vi "StorePreviousSwitchValues.vi"(0 "Array":u8[](array[numeric])) -> ()   [LabVIEW 2018]
uses:
  CurrentSwitchValues_GlobalVariable.vi
panel:
  out "30":dbl
  out "29":dbl
  out "28":dbl
  out "27":dbl
  out "26":dbl
  out "25":dbl
  out "24":dbl
  out "23":dbl
  out "22":dbl
  out "21":dbl
  out "20":dbl
  out "19":dbl
  out "18":dbl
  out "17":dbl
  out "16":dbl
  out "15":dbl
  out "14":dbl
  out "13":dbl
  out "12":dbl
  out "11":dbl
  out "10":dbl
  out "9":dbl
  out "8":dbl
  out "7":dbl
  out "6":dbl
  out "5":dbl
  out "4":dbl
  out "3":dbl
  out "2":dbl
  out "1":dbl
  out "[3]":string
  out "[4]":string
  out "[1]":string
  out "[2]":string
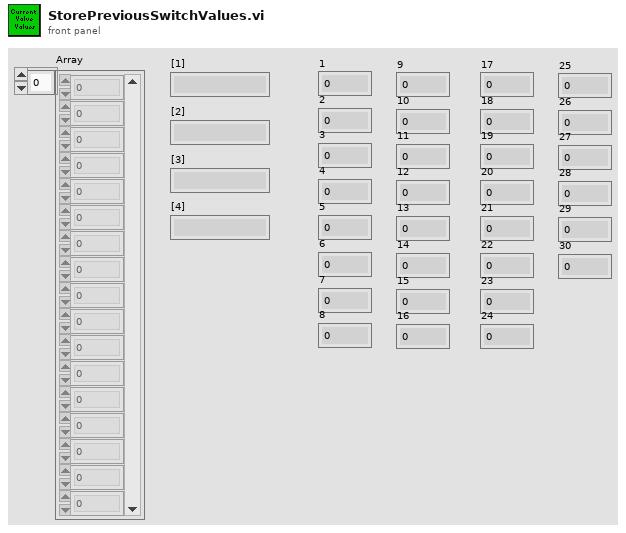
[diagram p1: front panel]
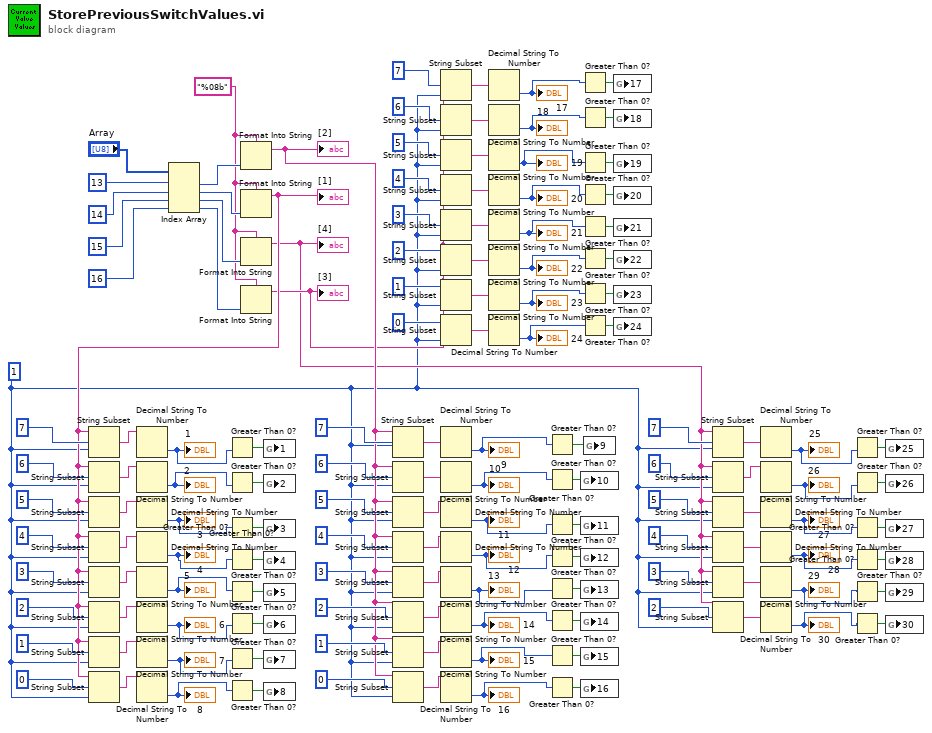
[diagram p0: block diagram]
diagram:
  w1 = 1
  w110 = "%08b"
  n1 = Index Array(array="Array", index #1=13, index #2=14, index #3=15, index #4=16) -> (element #1=w130:u8, element #2=w127:u8, element #3=w128:u8, element #4=w129:u8)
  n2 = Format Into String(format string=w110, w130) -> (resulting string=w93:string)  [unwired: 2 in, 1 out]
  "[2]" <- w93
  n3 = Format Into String(format string=w110, w127) -> (resulting string=w92:string)  [unwired: 2 in, 1 out]
  "[1]" <- w92
  n4 = String Subset(string=w92, offset (0)=7, length (rest)=w1) -> (substring=w126:string)
  n5 = String Subset(string=w92, offset (0)=6, length (rest)=w1) -> (substring=w119:string)
  n6 = String Subset(string=w92, offset (0)=5, length (rest)=w1) -> (substring=w120:string)
  n7 = String Subset(string=w92, offset (0)=4, length (rest)=w1) -> (substring=w121:string)
  n8 = String Subset(string=w92, offset (0)=3, length (rest)=w1) -> (substring=w122:string)
  n9 = String Subset(string=w92, offset (0)=2, length (rest)=w1) -> (substring=w123:string)
  n10 = String Subset(string=w92, offset (0)=1, length (rest)=w1) -> (substring=w124:string)
  n11 = String Subset(string=w92, offset (0)=0, length (rest)=w1) -> (substring=w125:string)
  n12 = Decimal String To Number(string=w126) -> (number=w61:i32)  [unwired: 2 in, 1 out]
  "1" <- w61
  n13 = Decimal String To Number(string=w119) -> (number=w46:i32)  [unwired: 2 in, 1 out]
  "2" <- w46
  n14 = Decimal String To Number(string=w120) -> (number=w47:i32)  [unwired: 2 in, 1 out]
  "3" <- w47
  n15 = Decimal String To Number(string=w121) -> (number=w48:i32)  [unwired: 2 in, 1 out]
  "4" <- w48
  n16 = Decimal String To Number(string=w122) -> (number=w49:i32)  [unwired: 2 in, 1 out]
  "5" <- w49
  n17 = Decimal String To Number(string=w123) -> (number=w50:i32)  [unwired: 2 in, 1 out]
  "6" <- w50
  n18 = Decimal String To Number(string=w124) -> (number=w51:i32)  [unwired: 2 in, 1 out]
  "7" <- w51
  n19 = Decimal String To Number(string=w125) -> (number=w52:i32)  [unwired: 2 in, 1 out]
  "8" <- w52
  n20 = Greater Than 0?(x=w61) -> (x > 0?=w60:bool)
  n21 = Greater Than 0?(x=w46) -> (x > 0?=w59:bool)
  n22 = Greater Than 0?(x=w47) -> (x > 0?=w58:bool)
  n23 = Greater Than 0?(x=w48) -> (x > 0?=w57:bool)
  n24 = Greater Than 0?(x=w49) -> (x > 0?=w56:bool)
  n25 = Greater Than 0?(x=w50) -> (x > 0?=w55:bool)
  n26 = Greater Than 0?(x=w51) -> (x > 0?=w54:bool)
  n27 = Greater Than 0?(x=w52) -> (x > 0?=w53:bool)
  n28 = Format Into String(format string=w110, w128) -> (resulting string=w63:string)  [unwired: 2 in, 1 out]
  "[4]" <- w63
  n29 = Format Into String(format string=w110, w129) -> (resulting string=w75:string)  [unwired: 2 in, 1 out]
  "[3]" <- w75
  n30 = global write "CurrentSwitchValues_GlobalVariable.vi" "1"(w60) -> ()
  n31 = global write "CurrentSwitchValues_GlobalVariable.vi" "2"(w59) -> ()
  n32 = global write "CurrentSwitchValues_GlobalVariable.vi" "3"(w58) -> ()
  n33 = global write "CurrentSwitchValues_GlobalVariable.vi" "4"(w57) -> ()
  n34 = global write "CurrentSwitchValues_GlobalVariable.vi" "5"(w56) -> ()
  n35 = global write "CurrentSwitchValues_GlobalVariable.vi" "6"(w55) -> ()
  n36 = global write "CurrentSwitchValues_GlobalVariable.vi" "7"(w54) -> ()
  n37 = global write "CurrentSwitchValues_GlobalVariable.vi" "8"(w53) -> ()
  n38 = String Subset(string=w93, offset (0)=7, length (rest)=w1) -> (substring=w109:string)
  n39 = String Subset(string=w93, offset (0)=6, length (rest)=w1) -> (substring=w102:string)
  n40 = String Subset(string=w93, offset (0)=5, length (rest)=w1) -> (substring=w103:string)
  n41 = String Subset(string=w93, offset (0)=4, length (rest)=w1) -> (substring=w104:string)
  n42 = String Subset(string=w93, offset (0)=3, length (rest)=w1) -> (substring=w105:string)
  n43 = String Subset(string=w93, offset (0)=2, length (rest)=w1) -> (substring=w106:string)
  n44 = String Subset(string=w93, offset (0)=1, length (rest)=w1) -> (substring=w107:string)
  n45 = String Subset(string=w93, offset (0)=0, length (rest)=w1) -> (substring=w108:string)
  n46 = String Subset(string=w75, offset (0)=7, length (rest)=w1) -> (substring=w91:string)
  n47 = String Subset(string=w75, offset (0)=6, length (rest)=w1) -> (substring=w84:string)
  n48 = String Subset(string=w75, offset (0)=5, length (rest)=w1) -> (substring=w85:string)
  n49 = String Subset(string=w75, offset (0)=4, length (rest)=w1) -> (substring=w86:string)
  n50 = String Subset(string=w75, offset (0)=3, length (rest)=w1) -> (substring=w87:string)
  n51 = String Subset(string=w75, offset (0)=2, length (rest)=w1) -> (substring=w88:string)
  n52 = String Subset(string=w75, offset (0)=1, length (rest)=w1) -> (substring=w89:string)
  n53 = String Subset(string=w75, offset (0)=0, length (rest)=w1) -> (substring=w90:string)
  n54 = Decimal String To Number(string=w109) -> (number=w21:i32)  [unwired: 2 in, 1 out]
  "9" <- w21
  n55 = Decimal String To Number(string=w102) -> (number=w20:i32)  [unwired: 2 in, 1 out]
  "10" <- w20
  n56 = Decimal String To Number(string=w103) -> (number=w19:i32)  [unwired: 2 in, 1 out]
  "11" <- w19
  n57 = Decimal String To Number(string=w104) -> (number=w18:i32)  [unwired: 2 in, 1 out]
  "12" <- w18
  n58 = Decimal String To Number(string=w105) -> (number=w17:i32)  [unwired: 2 in, 1 out]
  "13" <- w17
  n59 = Decimal String To Number(string=w106) -> (number=w16:i32)  [unwired: 2 in, 1 out]
  "14" <- w16
  n60 = Decimal String To Number(string=w107) -> (number=w15:i32)  [unwired: 2 in, 1 out]
  "15" <- w15
  n61 = Decimal String To Number(string=w108) -> (number=w14:i32)  [unwired: 2 in, 1 out]
  "16" <- w14
  n62 = Decimal String To Number(string=w91) -> (number=w22:i32)  [unwired: 2 in, 1 out]
  "17" <- w22
  n63 = Decimal String To Number(string=w84) -> (number=w23:i32)  [unwired: 2 in, 1 out]
  "18" <- w23
  n64 = Decimal String To Number(string=w85) -> (number=w24:i32)  [unwired: 2 in, 1 out]
  "19" <- w24
  n65 = Decimal String To Number(string=w86) -> (number=w25:i32)  [unwired: 2 in, 1 out]
  "20" <- w25
  n66 = Decimal String To Number(string=w87) -> (number=w26:i32)  [unwired: 2 in, 1 out]
  "21" <- w26
  n67 = Decimal String To Number(string=w88) -> (number=w27:i32)  [unwired: 2 in, 1 out]
  "22" <- w27
  n68 = Decimal String To Number(string=w89) -> (number=w28:i32)  [unwired: 2 in, 1 out]
  "23" <- w28
  n69 = Decimal String To Number(string=w90) -> (number=w29:i32)  [unwired: 2 in, 1 out]
  "24" <- w29
  n70 = Greater Than 0?(x=w21) -> (x > 0?=w38:bool)
  n71 = Greater Than 0?(x=w20) -> (x > 0?=w39:bool)
  n72 = Greater Than 0?(x=w19) -> (x > 0?=w40:bool)
  n73 = Greater Than 0?(x=w18) -> (x > 0?=w41:bool)
  n74 = Greater Than 0?(x=w17) -> (x > 0?=w42:bool)
  n75 = Greater Than 0?(x=w16) -> (x > 0?=w43:bool)
  n76 = Greater Than 0?(x=w15) -> (x > 0?=w44:bool)
  n77 = Greater Than 0?(x=w14) -> (x > 0?=w45:bool)
  n78 = Greater Than 0?(x=w22) -> (x > 0?=w37:bool)
  n79 = Greater Than 0?(x=w23) -> (x > 0?=w36:bool)
  n80 = Greater Than 0?(x=w24) -> (x > 0?=w35:bool)
  n81 = Greater Than 0?(x=w25) -> (x > 0?=w34:bool)
  n82 = Greater Than 0?(x=w26) -> (x > 0?=w33:bool)
  n83 = Greater Than 0?(x=w27) -> (x > 0?=w32:bool)
  n84 = Greater Than 0?(x=w28) -> (x > 0?=w31:bool)
  n85 = Greater Than 0?(x=w29) -> (x > 0?=w30:bool)
  n86 = global write "CurrentSwitchValues_GlobalVariable.vi" "10"(w39) -> ()
  n87 = global write "CurrentSwitchValues_GlobalVariable.vi" "11"(w40) -> ()
  n88 = global write "CurrentSwitchValues_GlobalVariable.vi" "12"(w41) -> ()
  n89 = global write "CurrentSwitchValues_GlobalVariable.vi" "13"(w42) -> ()
  n90 = global write "CurrentSwitchValues_GlobalVariable.vi" "14"(w43) -> ()
  n91 = global write "CurrentSwitchValues_GlobalVariable.vi" "15"(w44) -> ()
  n92 = global write "CurrentSwitchValues_GlobalVariable.vi" "16"(w45) -> ()
  n93 = global write "CurrentSwitchValues_GlobalVariable.vi" "9"(w38) -> ()
  n94 = global write "CurrentSwitchValues_GlobalVariable.vi" "17"(w37) -> ()
  n95 = global write "CurrentSwitchValues_GlobalVariable.vi" "18"(w36) -> ()
  n96 = global write "CurrentSwitchValues_GlobalVariable.vi" "19"(w35) -> ()
  n97 = global write "CurrentSwitchValues_GlobalVariable.vi" "20"(w34) -> ()
  n98 = global write "CurrentSwitchValues_GlobalVariable.vi" "21"(w33) -> ()
  n99 = global write "CurrentSwitchValues_GlobalVariable.vi" "22"(w32) -> ()
  n100 = global write "CurrentSwitchValues_GlobalVariable.vi" "23"(w31) -> ()
  n101 = global write "CurrentSwitchValues_GlobalVariable.vi" "24"(w30) -> ()
  n102 = String Subset(string=w63, offset (0)=7, length (rest)=w1) -> (substring=w74:string)
  n103 = String Subset(string=w63, offset (0)=6, length (rest)=w1) -> (substring=w62:string)
  n104 = String Subset(string=w63, offset (0)=5, length (rest)=w1) -> (substring=w70:string)
  n105 = String Subset(string=w63, offset (0)=4, length (rest)=w1) -> (substring=w71:string)
  n106 = String Subset(string=w63, offset (0)=3, length (rest)=w1) -> (substring=w72:string)
  n107 = String Subset(string=w63, offset (0)=2, length (rest)=w1) -> (substring=w73:string)
  n108 = Decimal String To Number(string=w74) -> (number=w7:i32)  [unwired: 2 in, 1 out]
  "25" <- w7
  n109 = Decimal String To Number(string=w62) -> (number=w6:i32)  [unwired: 2 in, 1 out]
  "26" <- w6
  n110 = Decimal String To Number(string=w70) -> (number=w5:i32)  [unwired: 2 in, 1 out]
  "27" <- w5
  n111 = Decimal String To Number(string=w71) -> (number=w4:i32)  [unwired: 2 in, 1 out]
  "28" <- w4
  n112 = Decimal String To Number(string=w72) -> (number=w3:i32)  [unwired: 2 in, 1 out]
  "29" <- w3
  n113 = Decimal String To Number(string=w73) -> (number=w2:i32)  [unwired: 2 in, 1 out]
  "30" <- w2
  n114 = Greater Than 0?(x=w7) -> (x > 0?=w8:bool)
  n115 = Greater Than 0?(x=w6) -> (x > 0?=w9:bool)
  n116 = Greater Than 0?(x=w5) -> (x > 0?=w10:bool)
  n117 = Greater Than 0?(x=w4) -> (x > 0?=w11:bool)
  n118 = Greater Than 0?(x=w3) -> (x > 0?=w12:bool)
  n119 = Greater Than 0?(x=w2) -> (x > 0?=w13:bool)
  n120 = global write "CurrentSwitchValues_GlobalVariable.vi" "25"(w8) -> ()
  n121 = global write "CurrentSwitchValues_GlobalVariable.vi" "26"(w9) -> ()
  n122 = global write "CurrentSwitchValues_GlobalVariable.vi" "27"(w10) -> ()
  n123 = global write "CurrentSwitchValues_GlobalVariable.vi" "28"(w11) -> ()
  n124 = global write "CurrentSwitchValues_GlobalVariable.vi" "29"(w12) -> ()
  n125 = global write "CurrentSwitchValues_GlobalVariable.vi" "30"(w13) -> ()
